vi "consumer.vi"(7 "Cluster":T1, 8 "error in":errorcluster, 11 "queue in":refnum<queue>) -> (0 "error out":errorcluster, 1 "counter":i32)   [LabVIEW 2010]
uses:
  references.ctl
  <vilib>/Utility/error.llb/DialogType.ctl
  <vilib>/Utility/file.llb/Read From Spreadsheet File (string).vi
  <vilib>/Utility/file.llb/Write To Spreadsheet File (string).vi
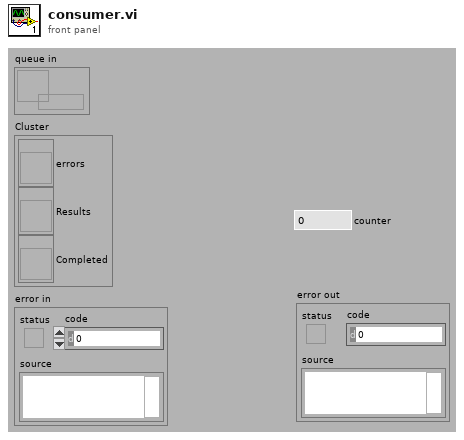
[diagram p1: front panel]
types:
  T1 = typedef "references.ctl" = cluster{"errors":refnum<vi>, "Results":refnum<vi>, "Completed":refnum<vi>}
  T2 = typedef "DialogType.ctl" = u16
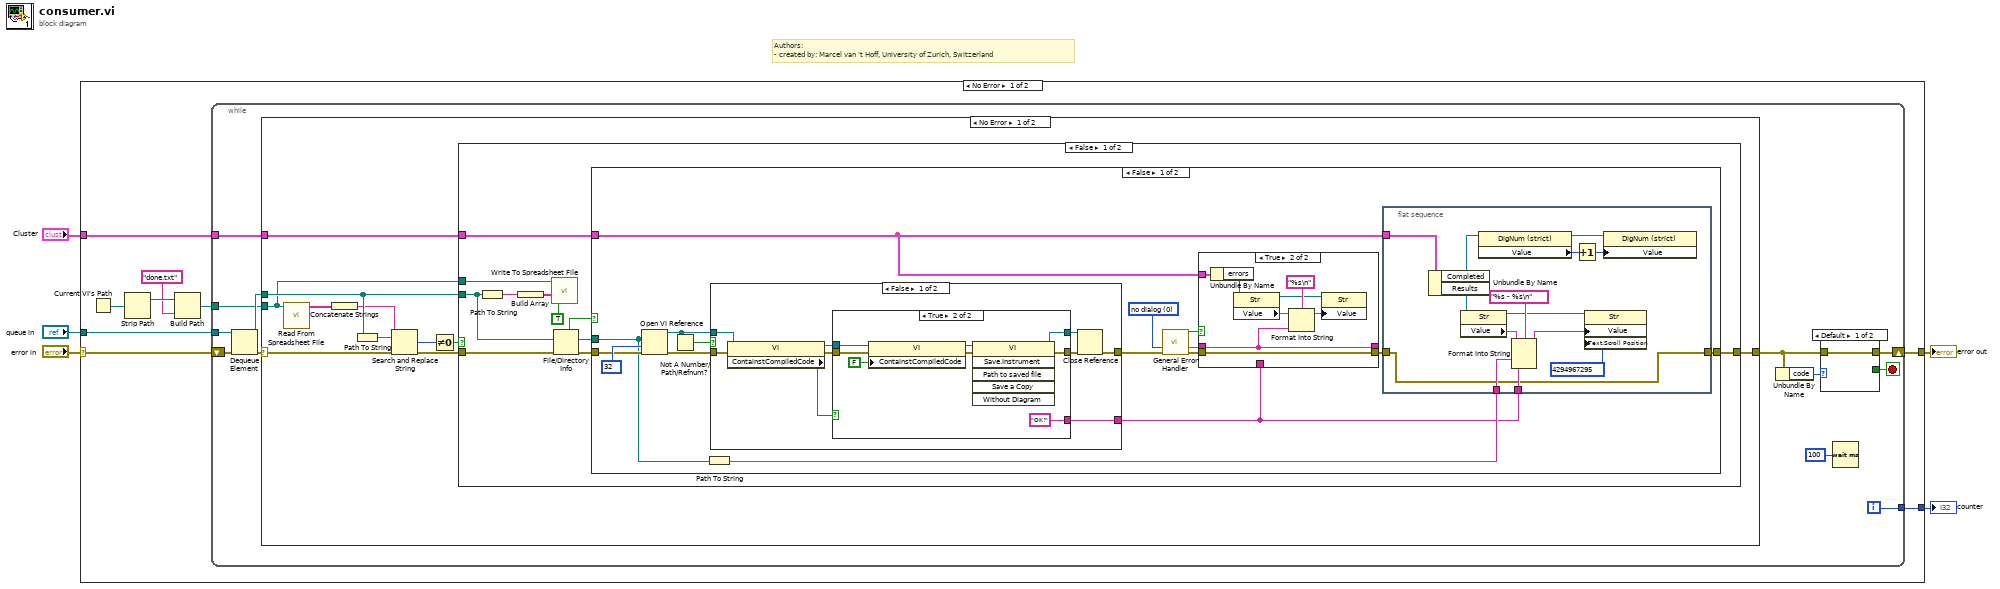
[diagram p0: block diagram]
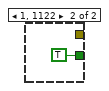
[diagram p2: hidden frame]
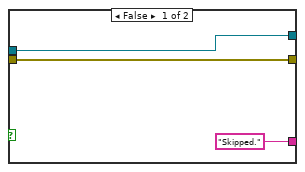
[diagram p4: hidden frame]
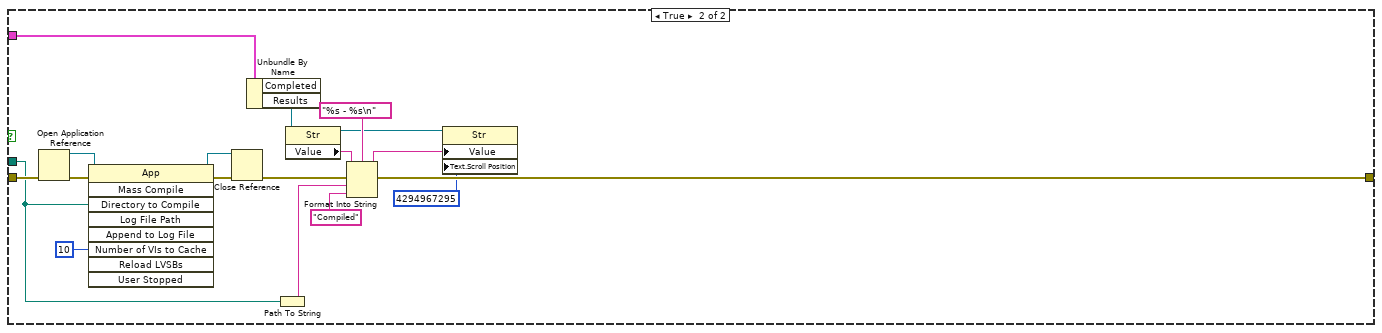
[diagram p6: hidden frame]
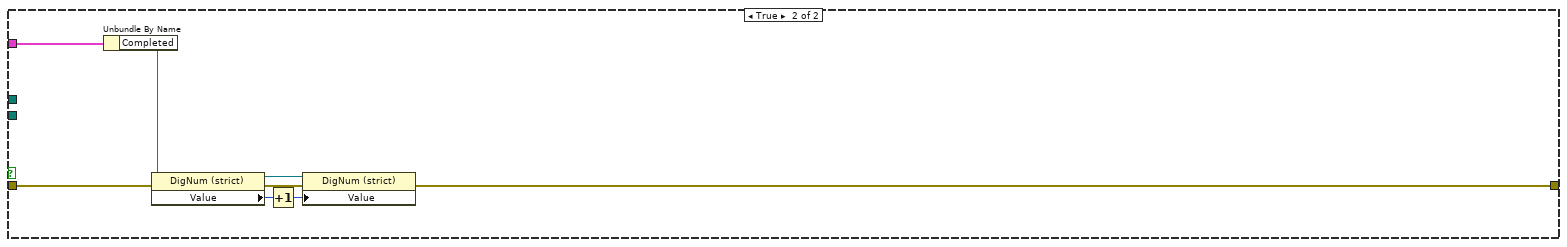
[diagram p7: hidden frame]
diagram:
  # "Authors: \n- created by: Marcel van 't Hoff, University of Zurich, Switzerland"
  n1 = case shown="No Error" "error in" {
    selector: "error in" -> [w6 w139]
    tunnel: "Cluster" -> [w14 _]
    tunnel: "queue in" -> [w13 _]
    tunnel: [w11 w139] -> w3
    tunnel: [w12 _] -> w1
    frame No Error {
      n2 = Current VI's Path() -> (path=w10:path)
      n3 = Strip Path(path=w10) -> (stripped path=w9:path)  [unwired: 1 out]
      n4 = Build Path(base path=w9, name or relative path="done.txt") -> (appended path=w7:path)
      n5 = while {
        tunnel: w13 -> [w26]
        tunnel: w14 -> [w23]
        tunnel: [w22] -> w12
        tunnel: w7 -> [w16]
        shift-right: [w18] -> w11
        shift-left: w6 -> [w15]
        i -> [w22]
        stop <- w19 stop-if-true
        n6 = Dequeue Element(queue=w26, error in (no error)=w15) -> (element=w25:path, error out=w24:errorcluster)  [unwired: 1 in, 2 out]
        n7 = case shown="No Error" w24 {
          selector: w24 -> [w31 w138]
          tunnel: w25 -> [w35 _]
          tunnel: [w39 w138] -> w20
          tunnel: w23 -> [w38 _]
          tunnel: w16 -> [w30 _]
          frame No Error {
            n8 = call-poly <vilib>:"Read From Spreadsheet File.vi"("file path (dialog if empty)"=w30) -> ("all rows"=w33:string[][])  [unwired: 6 in, 4 out]
            n9 = Concatenate Strings(w33) -> (w32:string)
            n10 = Path To String(path=w35) -> (string=w29:string)
            n11 = Search and Replace String(input string=w32, search string=w29, error in=w31) -> (number of replacements=w37:i32, error out=w36:errorcluster)  [unwired: 5 in, 2 out]
            n12 = Not Equal To 0?(x=w37) -> (x != 0?=w34:bool)
            n13 = case shown="False" w34 {
              tunnel: [w50 w130] -> w39
              tunnel: w38 -> [w49 w135]
              tunnel: w36 -> [w45 w131]
              tunnel: w35 -> [w44 _]
              tunnel: w30 -> [w40 _]
              frame False {
                n14 = Path To String(path=w44) -> (string=w43:string)
                n15 = Build Array(w43) -> (w42:string[])
                n16 = call-poly <vilib>:"Write To Spreadsheet File.vi"("append to file? (new file:F)"=TRUE, "1D data"=w42, "file path (dialog if empty)"=w40) -> ()  [unwired: 5 in, 1 out]
                n17 = File/Directory Info(path=w44, error in=w45) -> (path out=w47:path, directory=w48:bool, error out=w46:errorcluster)  [unwired: 4 out]
                n18 = case shown="False" w48 {
                  tunnel: w46 -> [w54 w124]
                  tunnel: [w53 w122] -> w50
                  tunnel: w49 -> [w52 w121]
                  tunnel: w47 -> [w51 w120]
                  frame False {
                    w61 = T2 0 items=["no dialog", "OK message", "continue or stop message", "OK message + warnings", "continue/stop + warnings"] ("type of dialog (OK msg:1)")
                    n19 = Open VI Reference(vi path=w51, options=32, error in (no error)=w54) -> (vi reference=w63:refnum<vi>, error out=w65:errorcluster)  [unwired: 3 in]
                    n20 = Not A Number/Path/Refnum?(number/path/refnum=w63) -> (NaN/Path/Refnum?=w64:bool)
                    n21 = Path To String(path=w51) -> (string=w56:string)
                    n22 = case shown="False" w64 {
                      tunnel: w63 -> [w94 _]
                      tunnel: w65 -> [w93 w111]
                      tunnel: [w99 w111] -> w62
                      tunnel: [w95 _] -> w55
                      frame False {
                        n23 = property class="VI"(reference=w94, error in=w93) -> (reference out=w91:refnum<vi>, error out=w92:errorcluster, "ContainstCompiledCode"=w96:bool)
                        n24 = case shown="True" w96 {
                          tunnel: w92 -> [w102 w109]
                          tunnel: w91 -> [w101 w108]
                          tunnel: [w102 w106] -> w98
                          tunnel: [w101 w105] -> w97
                          tunnel: ["Skipped." "OK!"] -> w95
                          frame False {
                          }
                          frame True {
                            n25 = property class="VI"(reference=w108, error in=w109, "ContainstCompiledCode"=FALSE ("Contains Compiled Code")) -> (reference out=w103:refnum<vi>, error out=w107:errorcluster)
                            n26 = invoke class="VI" method="Save.Instrument"(reference=w103, error in=w107) -> (reference out=w105:refnum<vi>, error out=w106:errorcluster)  [unwired: 4 in, 4 out]
                          }
                        }
                        n27 = Close Reference(reference=w97, error in (no error)=w98) -> (error out=w99:errorcluster)
                      }
                      frame True {
                      }
                    }
                    n28 = call <vilib>:"General Error Handler.vi"("type of dialog (OK msg:1)"=w61, "error in (no error)"=w62) -> ("error?"=w59:bool, "message"=w60:string, "error out"=w58:errorcluster)  [unwired: 9 in, 2 out]
                    n29 = case shown="True" w59 {
                      tunnel: [w82 w90] -> _
                      tunnel: w60 -> [_ w90]
                      tunnel: w55 -> [w82 _]
                      tunnel: w58 -> [w81 w83]
                      tunnel: [w81 w83] -> w57
                      tunnel: w52 -> [_ w88]
                      frame False {
                      }
                      frame True {
                        n30 = Unbundle By Name(w88) -> ("errors"=w87:refnum<vi>)
                        n31 = property class="Str"(reference=w87) -> (reference out=w84:refnum<vi>, "Value"=w86:string)  [unwired: 1 in, 1 out]
                        n32 = Format Into String(format string="%s\n", initial string=w86, w90) -> (resulting string=w85:string)  [unwired: 1 in, 1 out]
                        n33 = property class="Str"(reference=w84, "Value"=w85) -> ()  [unwired: 1 in, 2 out]
                      }
                    }
                    n34 = flat-sequence {
                      tunnel: w57 -> [w67]
                      tunnel: w56 -> [w79]
                      tunnel: w55 -> [w78]
                      tunnel: [w67] -> w53
                      tunnel: w52 -> [w77]
                      frame #0 {
                        n35 = Unbundle By Name(w77) -> ("Completed"=w72:refnum<vi>, "Results"=w76:refnum<vi>)
                        n36 = property class="Str"(reference=w76) -> (reference out=w73:refnum<vi>, "Value"=w75:string)  [unwired: 1 in, 1 out]
                        n37 = property class="DigNum (strict)"(reference=w72) -> (reference out=w71:refnum<vi>, "Value"=w70:i32)  [unwired: 1 in, 1 out]
                        n38 = Format Into String(format string="%s - %s\n", initial string=w75, w79, w78) -> (resulting string=w74:string)  [unwired: 1 in, 1 out]
                        n39 = Increment(x=w70) -> (x+1=w69:i32)
                        n40 = property class="Str"(reference=w73, "Value"=w74, "Text.Scroll Position"=u32 4294967295) -> ()  [unwired: 1 in, 2 out]
                        n41 = property class="DigNum (strict)"(reference=w71, "Value"=w69) -> ()  [unwired: 1 in, 2 out]
                      }
                    }
                  }
                  frame True {
                    n42 = Open Application Reference(8:w124) -> (0:w128:errorcluster, 3:w127:refnum<vi>)  [unwired: 3 in]
                    n43 = invoke class="App" method="Mass Compile"(reference=w127, error in=w128, "Directory to Compile"=w120, "Number of VIs to Cache"=u32 10) -> (reference out=w125:refnum<vi>, error out=w126:errorcluster)  [unwired: 5 in, 7 out]
                    n44 = Close Reference(reference=w125, error in (no error)=w126) -> (error out=w123:errorcluster)
                    n45 = Unbundle By Name(w121) -> ("Results"=w118:refnum<vi>)  [unwired: 1 out]
                    n46 = Path To String(path=w120) -> (string=w113:string)
                    n47 = property class="Str"(reference=w118) -> (reference out=w115:refnum<vi>, "Value"=w117:string)  [unwired: 1 in, 1 out]
                    n48 = Format Into String(format string="%s - %s\n", initial string=w117, error in=w123, w113, "Compiled" ("input 2")) -> (resulting string=w116:string, error out=w122:errorcluster)
                    n49 = property class="Str"(reference=w115, "Value"=w116, "Text.Scroll Position"=u32 4294967295) -> ()  [unwired: 1 in, 2 out]
                  }
                }
              }
              frame True {
                n50 = Unbundle By Name(w135) -> ("Completed"=w134:refnum<vi>)
                n51 = property class="DigNum (strict)"(reference=w134, error in=w131) -> (reference out=w132:refnum<vi>, error out=w133:errorcluster, "Value"=w137:i32)
                n52 = Increment(x=w137) -> (x+1=w136:i32)
                n53 = property class="DigNum (strict)"(reference=w132, error in=w133, "Value"=w136) -> (error out=w130:errorcluster)  [unwired: 1 out]
              }
            }
          }
          frame Error {
          }
        }
        n54 = Unbundle By Name(w20) -> ("code"=w21:i32)
        n55 = case shown="Default" w21 {
          tunnel: [w27 _] -> w18
          tunnel: w20 -> [w27 _]
          tunnel: [_ TRUE] -> w19
          frame Default {
          }
          frame 1, 1122 {
          }
        }
        n56 = Wait (ms)(milliseconds to wait=u32 100) -> ()  [unwired: 1 out]
      }
    }
    frame Error {
    }
  }
  "error out" <- w3
  "counter" <- w1
